vi "CurrentInstance.vi"(11 "error in (no error)":errorcluster) -> (15 "error out":errorcluster)   [LabVIEW 2016, in "DronaTest.lvlib"]
uses:
  DronaTest.lvlib
  APIs/Get/GetVI/GetVIByPath.vi
  APIs/Stimulus/VI/RunVI.vi
  APIs/Stimulus/VI/MakeVIFrontMost.vi
  Drona.lvlib
  APIs/Get/GetVI/GetVI.lvlib
  <vilib>/addons/_JKI Toolkits/Caraya/classes/Test/Test.lvclass
  APIs/Stimulus/VI/VI.lvlib
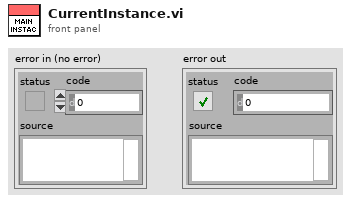
[diagram p1: front panel]
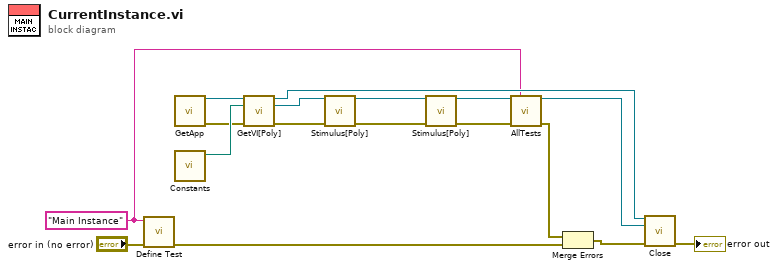
[diagram p0: block diagram]
diagram:
  w3 = "Main Instance" ("Label (VI Title)")
  n1 = call <vilib>:"Define Test.vi"("error in (no error)"="error in (no error)", "Label (VI Title)"=w3) -> ("error out"=w6:errorcluster)  [unwired: 9 in]
  n2 = call "GetApp.vi"() -> ("Application Ref"=w9:refnum<vi>, "error out"=w8:errorcluster)  [unwired: 14 in]
  n3 = call "Constants.vi"() -> ("HelperMain path"=w17:path)  [unwired: 5 in, 6 out]
  n4 = call-poly "GetVI[Poly].vi"("Application Ref in"=w9, "VI Path"=w17, "error in (no error)"=w8) -> ("Application Ref out"=w4:refnum<vi>, "VI Reference"=w10:refnum<vi>, "error out"=w11:errorcluster)  [unwired: 10 in]
  n5 = call-poly "Stimulus[Poly].vi"("VI Reference In"=w10, "error in"=w11) -> ("VI Reference Out"=w15:refnum<vi>, "error out"=w16:errorcluster)  [unwired: 12 in]
  n6 = call-poly "Stimulus[Poly].vi"("VI Reference In"=w15, "error in"=w16) -> ("VI Reference Out"=w13:refnum<vi>, "error out"=w12:errorcluster)  [unwired: 12 in]
  n7 = call "AllTests.vi"("VI in"=w13, "Label"=w3, "error in (no error)"=w12) -> ("VI out"=w14:refnum<vi>, "error out"=w5:errorcluster)  [unwired: 11 in]
  n8 = Merge Errors(w5, w6) -> (w2:errorcluster)
  n9 = call "Close.vi"("Application Ref"=w4, "VI Reference"=w14, "error in"=w2) -> ("error out"=→"error out":errorcluster)  [unwired: 12 in]
